vi "Go to localize.vi"(8 "error in (no error)":errorcluster, 11 "States.lvlib:Localize.lvclass":refnum<class "Localize.lvclass">) -> (0 "error out":errorcluster, 3 "Process State out":refnum<class "State Actor.lvclass">)   [LabVIEW 2014, in "States.lvlib" / "Localize.lvclass"]
uses:
  Localize.lvclass
  <vilib>/NI/Actors/State Actor/State Actor/State Actor.lvclass
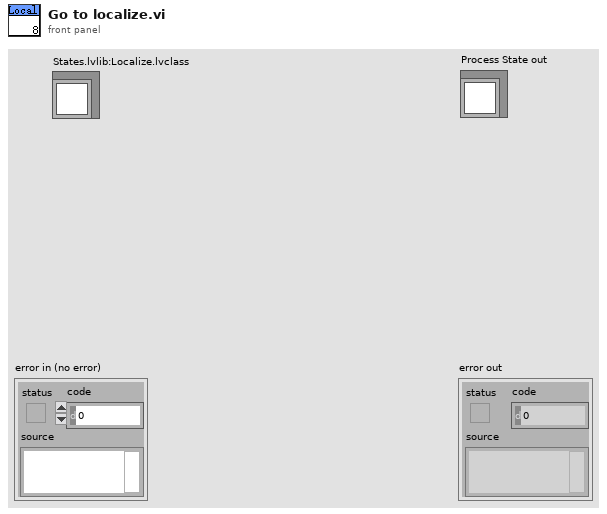
[diagram p1: front panel]
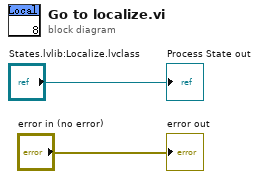
[diagram p0: block diagram]
diagram:
  "error out" <- "error in (no error)"
  "Process State out" <- "States.lvlib:Localize.lvclass"
